vi "Prober_CloseSession.vi"(8 "error in (no error)":errorcluster, 11 "TeslaVeloxProbeStation in":refnum<class "TeslaVeloxProbeStation.lvclass">) -> (0 "error out":errorcluster, 3 "TeslaVeloxProbeStation out":refnum<class "TeslaVeloxProbeStation.lvclass">)   [LabVIEW 2018, in "TeslaVeloxProbeStation.lvclass"]
uses:
  TeslaVeloxProbeStation.lvclass
  <instrlib>/CascadeProbestation/CascadeProbestation.lvlib
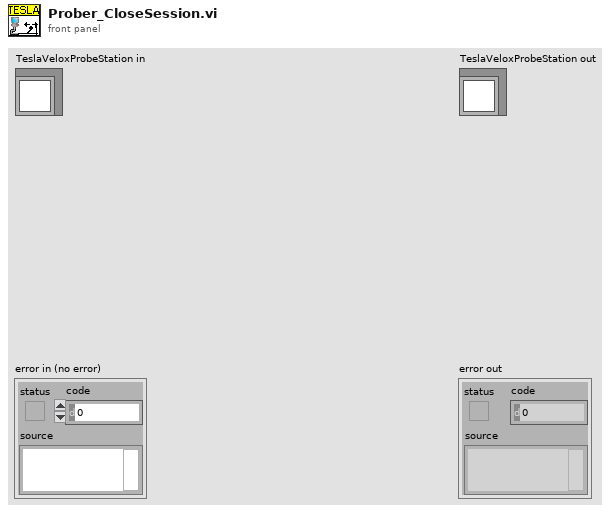
[diagram p1: front panel]
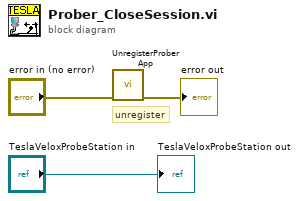
[diagram p0: block diagram]
diagram:
  # "unregister"
  n1 = call <instrlib>:"UnregisterProberApp.vi"("Error In"="error in (no error)") -> ("Error Out"=→"error out":errorcluster)  [unwired: 10 in]
  "TeslaVeloxProbeStation out" <- "TeslaVeloxProbeStation in"
